vi "Transceiver Receive.vi"(8 "error in (no error)":errorcluster, 10 "Transfer Group in":refnum<class "Transfer Group.lvclass">, 11 "Transceiver Thread in":refnum<class "Transceiver Thread.lvclass">) -> (0 "error out":errorcluster, 2 "Transfer Group out":refnum<class "Transfer Group.lvclass">, 3 "Transceiver Thread out":refnum<class "Transceiver Thread.lvclass">)   [LabVIEW 2017, in "DSF Core.lvlib" / "Transceiver Thread.lvclass"]
uses:
  Transceiver Thread.lvclass
  Transfer Group/Transfer Group.lvclass
  Transceiver Thread.lvclass/Transceiver Thread.ctl
  Transceiver/Transceiver.lvclass
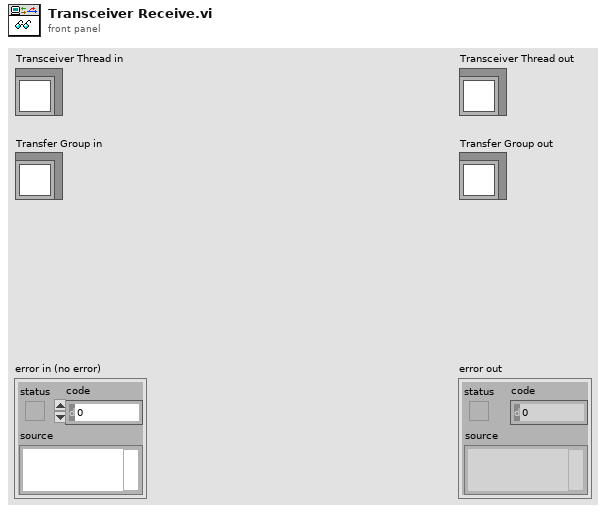
[diagram p1: front panel]
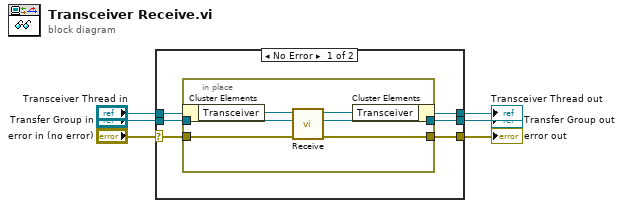
[diagram p0: block diagram]
diagram:
  n1 = case shown="No Error" "error in (no error)" {
    selector: "error in (no error)" -> [w7 w21]
    tunnel: "Transfer Group in" -> [w12 w19]
    tunnel: "Transceiver Thread in" -> [w11 w20]
    tunnel: [w10 w20] -> w4
    tunnel: [w9 w19] -> w3
    tunnel: [w8 w21] -> w2
    frame No Error {
      n2 = in-place {
        in-place-border: w7 -> [w16]
        in-place-border: w12 -> [w14]
        in-place-border: [w15] -> w8
        in-place-border: [w13] -> w9
        n3 = in-place-cluster #1(w11) -> ("Transceiver"=w18:refnum<class "Transceiver.lvclass">)
        n4 = call-dynamic "Receive.vi"("error in (no error)"=w16, "Transfer Group in"=w14, "Transceiver in"=w18) -> ("error out"=w15:errorcluster, "Transfer Group out"=w13:refnum<class "Transfer Group.lvclass">, "Transceiver out"=w17:refnum<class "Transceiver.lvclass">)  [unwired: 6 in]
        n5 = in-place-cluster #1("Transceiver"=w17) -> (w10:refnum<class "Transceiver Thread.lvclass">)
      }
    }
    frame Error {
    }
  }
  "error out" <- w2
  "Transceiver Thread out" <- w4
  "Transfer Group out" <- w3
